vi "FilterOnNameInTree.vi"() -> ()   [LabVIEW 2013]
doc: "Provides a mechanism to allow the user to specify a string to be searched for. Tree items containing a match continue to be displayed, while all non-matching items are removed from the tree. Also, a count of matching tree items is displayed, along with a count of all tree items."
uses:
  <vilib>/Utility/miscctls.llb/LVSelectionTypeDef.ctl
  FindName Task_Manager.lvlib
panel:
  out "Found/Total =":string
  in  "Data Tree":refnum<vi>
  in  "NameToFilter":string caption="Filter ="
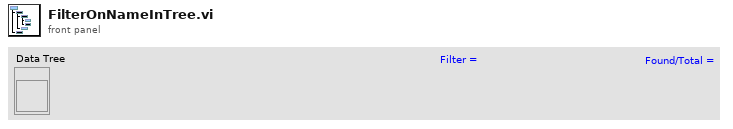
[diagram p1: front panel]
types:
  T1 = typedef "LVSelectionTypeDef.ctl" = cluster{"Selection Start":u32, "Selection End":u32}
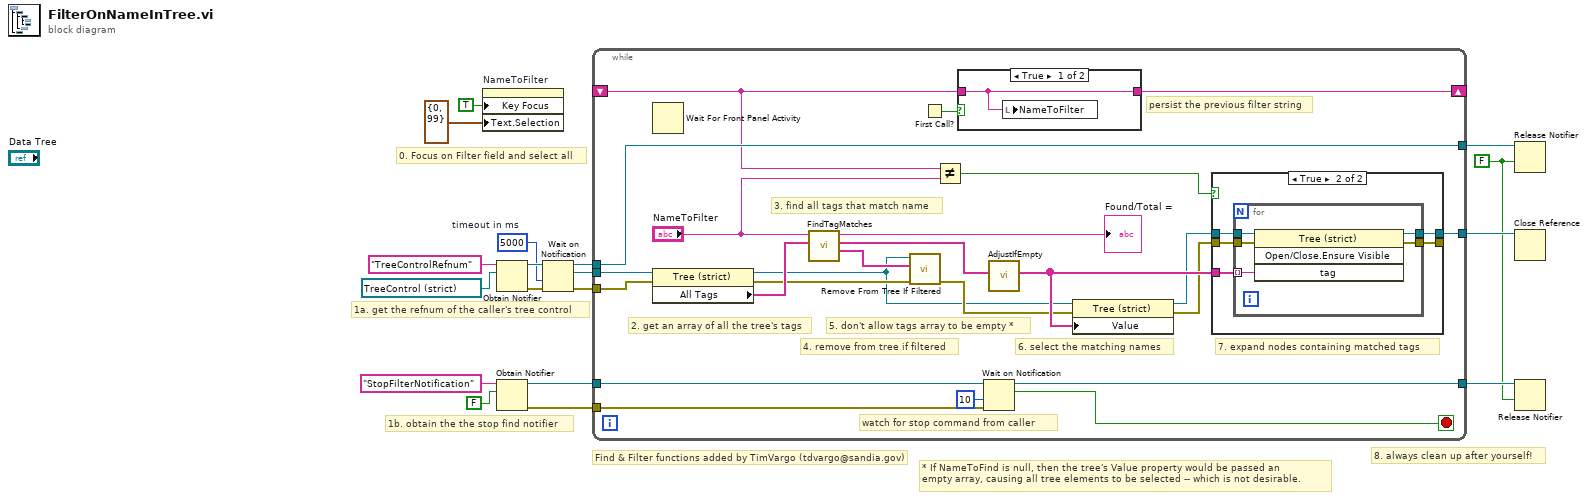
[diagram p0: block diagram]
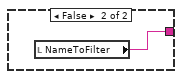
[diagram p3: hidden frame]
diagram:
  w1 = FALSE ("force destroy? (F)")
  w5 = 5000  # timeout in ms
  # "Find & Filter functions added by TimVargo (tdvargo@sandia.gov)"
  # "* If NameToFind is null, then the tree's Value property would be passed an \nempty array, causing all tree elements to be selected -- which is not desirable."
  # "1b. obtain the the stop find notifier"
  # "0. Focus on Filter field and select all"
  # "8. always clean up after yourself!"
  # "1a. get the refnum of the caller's tree control"
  n1 = property on="NameToFilter" class="Str"("Key Focus"=TRUE, "Text.Selection"=T1 {"Selection Start"=0, "Selection End"=99}) -> ()  [unwired: 2 in, 2 out]
  n2 = Obtain Notifier(name (unnamed)="TreeControlRefnum", notification data type=refnum<vi> refnum ("Data Tree")) -> (notifier out=w15:refnum<notifier>, error out=w16:errorcluster)  [unwired: 2 in, 1 out]
  n3 = Obtain Notifier(name (unnamed)="StopFilterNotification", notification data type=FALSE) -> (notifier out=w4:refnum<notifier>, error out=w3:errorcluster)  [unwired: 2 in, 1 out]
  n4 = Wait on Notification(notifier=w15, timeout in ms (-1)=w5, error in (no error)=w16) -> (notifier out=w13:refnum<notifier>, notification=w14:refnum<vi>, error out=w10:errorcluster)  [unwired: 1 in, 1 out]
  n5 = while {
    tunnel: w14 -> [w41]
    tunnel: w13 -> [w40]
    tunnel: [w40] -> w12
    tunnel: [w26] -> w11
    tunnel: w10 -> [w24]
    shift-right: [w38] -> _
    shift-left: _ -> [w25]
    tunnel: w4 -> [w36]
    tunnel: w3 -> [w35]
    tunnel: [w34] -> w2
    stop <- w31 stop-if-true
    # "4. remove from tree if filtered"
    # "7. expand nodes containing matched tags"
    # "5. don't allow tags array to be empty *"
    # "watch for stop command from caller"
    # "persist the previous filter string"
    # "3. find all tags that match name"
    # "6. select the matching names"
    # "2. get an array of all the tree's tags"
    n6 = Wait For Front Panel Activity() -> ()  [unwired: 3 in, 1 out]
    n7 = property class="Tree (strict)"(reference=w41, error in=w24) -> (reference out=w20:refnum<vi>, error out=w21:errorcluster, "All Tags"=w37:string[])
    n8 = call "FindTagMatches.vi"("All Tags"=w37, "NameToFind"="NameToFilter") -> ("Not Found"=w23:string[], "Found"=w19:string[], "ResultString"=→"Found/Total =":string)  [unwired: 7 in]
    n9 = call "Remove From Tree If Filtered.vi"("error in (no error)"=w21, "Not Found"=w23, "TreeControl in"=w20) -> ("error out"=w22:errorcluster)  [unwired: 8 in]
    n10 = First Call?() -> (First Call?: T/F=w39:bool)
    n11 = Not Equal?(x=w25, y="NameToFilter") -> (x != y?=w29:bool)
    n12 = case shown="True" w39 {
      tunnel: [w55 w56] -> w38
      tunnel: w25 -> [w55 _]
      frame True {
        n13 = local write "NameToFilter"(w55) -> ()
      }
      frame False {
        n14 = local read "NameToFilter"() -> (w56:string)
      }
    }
    n15 = Wait on Notification(notifier=w36, timeout in ms (-1)=10, error in (no error)=w35) -> (notifier out=w34:refnum<notifier>, notification=w31:bool)  [unwired: 1 in, 2 out]
    n16 = call "AdjustIfEmpty.vi"("Found"=w19) -> ("FoundAdj"=w32:string[])  [unwired: 10 in]
    n17 = property class="Tree (strict)"(reference=w20, error in=w22, "Value"=w32) -> (reference out=w28:refnum<vi>, error out=w27:errorcluster)
    n18 = case shown="True" w29 {
      tunnel: [w43 w49] -> _
      tunnel: w27 -> [w43 w48]
      tunnel: w28 -> [w44 w47]
      tunnel: [w44 w46] -> w26
      tunnel: w32 -> [_ w45]
      frame False {
      }
      frame True {
        n19 = for {
          tunnel: [w54] -> w49
          tunnel: w48 -> [w53]
          tunnel: w47 -> [w52]
          tunnel: [w51] -> w46
          tunnel: w45 -> [w50] mode=indexing
          n20 = invoke class="Tree (strict)" method="Open/Close.Ensure Visible"(reference=w52, error in=w53, "tag"=w50) -> (reference out=w51:refnum<vi>, error out=w54:errorcluster)  [unwired: 1 in, 2 out]
        }
      }
    }
  }
  n21 = Release Notifier(notifier=w12, force destroy? (F)=w1) -> ()  [unwired: 1 in, 3 out]
  n22 = Close Reference(reference=w11) -> ()  [unwired: 1 in, 1 out]
  n23 = Release Notifier(notifier=w2, force destroy? (F)=w1) -> ()  [unwired: 1 in, 3 out]
